vi "Obtain Waveform Sessions.vi"(8 "error in":errorcluster, 10 "Result Wfm Data Refs":T1[](array[typedef]), 11 "Source Wfm Data Refs":T1[](array[typedef])) -> (0 "error out":errorcluster, 2 "Result Wfm Sessions":refnum<class "Single Waveform Read (DBL).lvclass">[](array[class]), 3 "Source Wfm Sessions":refnum<class "Single Waveform Read (DBL).lvclass">[](array[class]))   [LabVIEW 2014, in "Waveform-Processing-Custom-Device Engine.lvlib"]
uses:
  Waveform-Processing-Custom-Device Engine.lvlib
  <vilib>/NI Veristand/Custom Device API/Waveform Data Reference.ctl
  <vilib>/NI Veristand/Custom Device Waveform API/Single Waveform Read (DBL)/Single Waveform Read (DBL).lvclass
  <vilib>/NI Veristand/Custom Device Waveform API/Single Waveform Read (DBL)/NI VeriStand - Open Single Waveform Read Session (DBL).vi
  <vilib>/NI Veristand/Custom Device Waveform API/NI_VS Custom Device Waveform API.lvlib
  <vilib>/NI Veristand/Custom Device API/Custom Device API.lvlib
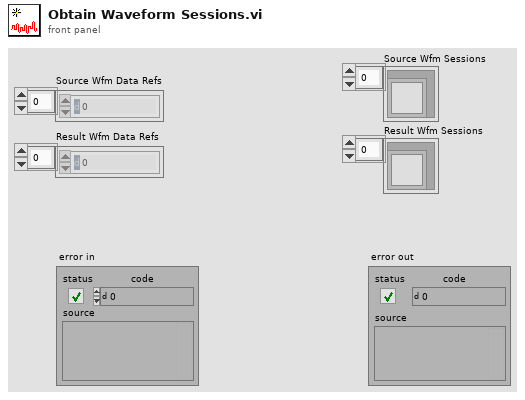
[diagram p1: front panel]
types:
  T1 = typedef "Custom Device API.lvlib/Waveform Data Reference.ctl" = i32
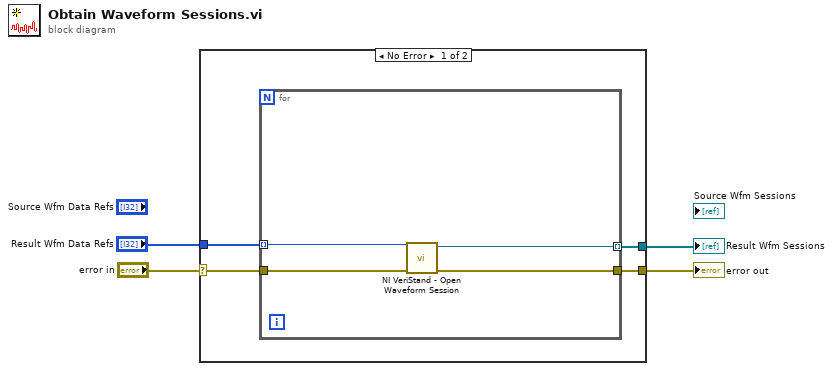
[diagram p0: block diagram]
diagram:
  n1 = case shown="No Error" "error in" {
    selector: "error in" -> [w8 w13]
    tunnel: [w5 w13] -> w3
    tunnel: "Result Wfm Data Refs" -> [w7 _]
    tunnel: [w6 _] -> w1
    frame No Error {
      n2 = for {
        tunnel: w8 -> [w12]
        tunnel: w7 -> [w11] mode=indexing
        tunnel: [w10] -> w6 mode=indexing
        tunnel: [w9] -> w5
        n3 = call-poly <vilib>:"NI VeriStand - Open Waveform Session.vi"("error in (no error)"=w12, "DBL Waveform Data Reference"=w11) -> ("error out"=w9:errorcluster, "Single Waveform Read Session (DBL)"=w10:refnum<class "Single Waveform Read (DBL).lvclass">)  [unwired: 8 in]
      }
    }
    frame Error {
    }
  }
  "error out" <- w3
  "Result Wfm Sessions" <- w1
